vi "tutorial_08.vi"() -> ()   [LabVIEW 2021]
uses:
  <vilib>/numeric/Random Number (Range) U64.vi
  <vilib>/numeric/sub_Random U32.vi
panel:
  in  "upper bound (100)":u64=100
  out "# interactions":dbl
  out "Current Number":dbl
  in  "Number to match":dbl
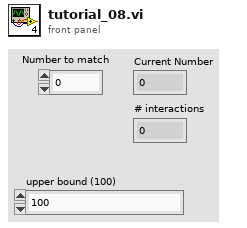
[diagram p1: front panel]
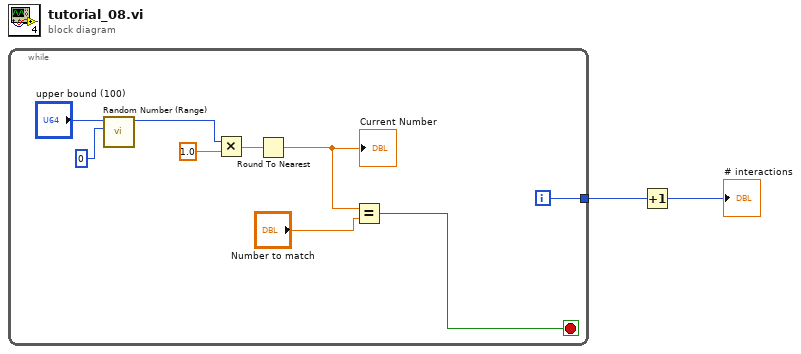
[diagram p0: block diagram]
diagram:
  n1 = while {
    tunnel: [w3] -> w1
    i -> [w3]
    stop <- w4 stop-if-true
    n2 = call-poly <vilib>:"Random Number (Range).vi"("lower bound (0)"=u64 0, "upper bound (100)"="upper bound (100)") -> ("number"=w10:u64)  [unwired: 9 in]
    n3 = Multiply(x=w10, y=1.0) -> (x*y=w9:dbl)
    n4 = Round To Nearest(number=w9) -> (nearest integer value=w5:dbl)
    "Current Number" <- w5
    n5 = Equal?(x=w5, y="Number to match") -> (x = y?=w4:bool)
  }
  n6 = Increment(x=w1) -> (x+1=→"# interactions":i32)
